vi "Read FixationRadius.vi"(8 "error in (no error)":errorcluster, 11 "BehaviorClassification in":refnum<class "BehaviorClassification.lvclass">) -> (0 "error out":errorcluster, 2 "FixationRadius":dbl, 3 "BehaviorClassification out":refnum<class "BehaviorClassification.lvclass">)   [LabVIEW 2010, in "BehaviorClassification.lvclass"]
uses:
  BehaviorClassification.lvclass
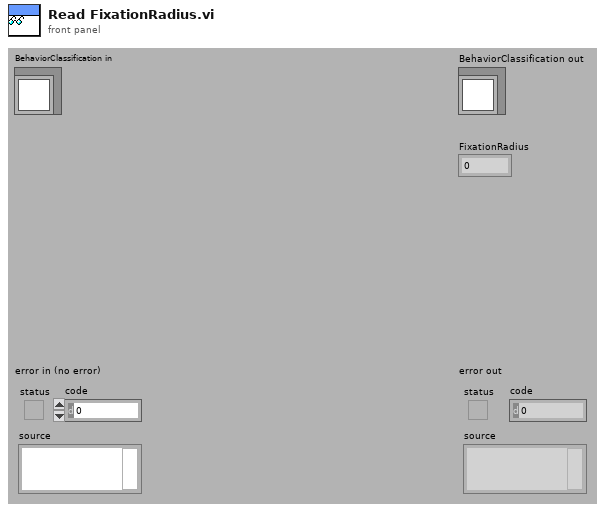
[diagram p1: front panel]
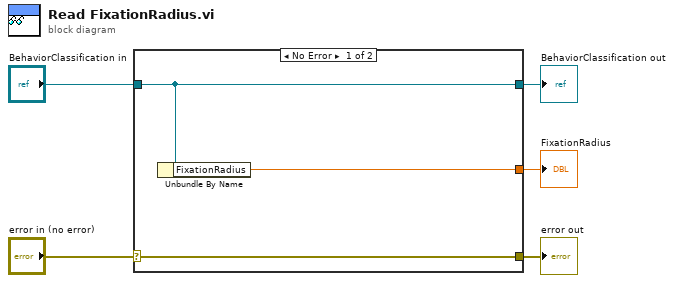
[diagram p0: block diagram]
diagram:
  n1 = case shown="No Error" "error in (no error)" {
    selector: "error in (no error)" -> [w8 w9]
    tunnel: [w8 w9] -> w4
    tunnel: [w7 w10] -> w2
    tunnel: "BehaviorClassification in" -> [w7 w10]
    tunnel: [w6 _] -> w1
    frame No Error {
      n2 = Unbundle By Name(w7) -> ("FixationRadius"=w6:dbl)
    }
    frame Error {
    }
  }
  "error out" <- w4
  "BehaviorClassification out" <- w2
  "FixationRadius" <- w1
